vi "ISX3_Cmd_SetSetupAddFrequencyEx.vi"(1 "Use LogScale":bool, 3 "PointDelay [µs]":u32, 5 "Start Frequency [Hz]":sgl=0.01 min=0.01 max=1e+07, 7 "Stop Frequency [Hz]":sgl=0.01 min=0.01 max=1e+07, 9 "Frequency Count":sgl=1.0 min=1 max=2048 step=1, 12 "Precision":sgl min=0, 13 "Amplitude [V]":sgl=0.01 min=0.001 max=1) -> (10 "set Setup Init Cmd":u8[](array[numeric]) format="%x")   [LabVIEW 2012, in "Sciospec ISX3 Impedance Analyzer.lvlib"]
uses:
  Sciospec ISX3 Impedance Analyzer.lvlib
panel:
  in  "Use PhaseSync":bool
  # "This VI generates the command to initate a new frequency block in the system with the PhaseSync and PointDelay option"
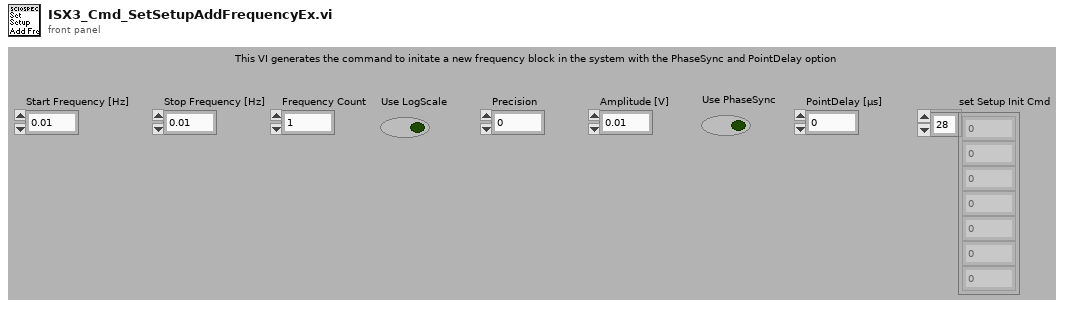
[diagram p1: front panel]
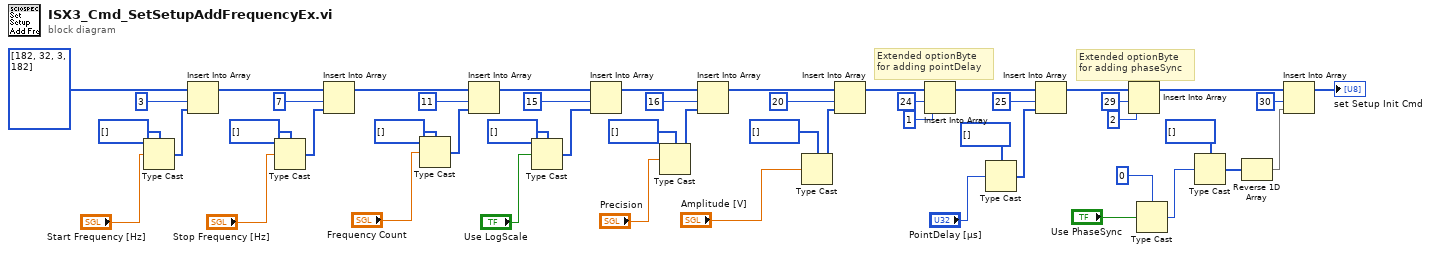
[diagram p0: block diagram]
diagram:
  # "Extended optionByte\nfor adding phaseSync"
  # "Extended optionByte\nfor adding pointDelay"
  n1 = Type Cast(type=u8[] [], x="Start Frequency [Hz]") -> (*(type *) &x=w47:u8[])
  n2 = Insert Into Array(array=u8[] [182, 32, 3, 182], index=3, new element=w47) -> (w45:u8[])
  n3 = Type Cast(type=u8[] [], x="Stop Frequency [Hz]") -> (*(type *) &x=w40:u8[])
  n4 = Insert Into Array(array=w45, index=7, new element=w40) -> (w24:u8[])
  n5 = Type Cast(type=u8[] [], x="Frequency Count") -> (*(type *) &x=w26:u8[])
  n6 = Insert Into Array(array=w24, index=11, new element=w26) -> (w23:u8[])
  n7 = Type Cast(type=u8[] [], x="Use LogScale") -> (*(type *) &x=w37:u8[])
  n8 = Insert Into Array(array=w23, index=15, new element=w37) -> (w44:u8[])
  n9 = Type Cast(type=u8[] [], x="Precision") -> (*(type *) &x=w34:u8[])
  n10 = Insert Into Array(array=w44, index=16, new element=w34) -> (w43:u8[])
  n11 = Type Cast(type=u8[] [], x="Amplitude [V]") -> (*(type *) &x=w30:u8[])
  n12 = Insert Into Array(array=w43, index=20, new element=w30) -> (w20:u8[])
  n13 = Insert Into Array(array=w20, index=24 ("Index"), new element=u8 1 ("Neues Element/Teil-Array")) -> (w10:u8[])
  n14 = Type Cast(type=u8[] [], x="PointDelay [µs]") -> (*(type *) &x=w8:u8[])
  n15 = Insert Into Array(array=w10, index=25 ("Index"), new element=w8) -> (w6:u8[])
  n16 = Insert Into Array(array=w6, index=29 ("Index"), new element=u8 2 ("Neues Element/Teil-Array")) -> (w15:u8[])
  n17 = Type Cast(type=u32 0, x="Use PhaseSync") -> (*(type *) &x=w3:u32)
  n18 = Type Cast(type=u8[] [], x=w3) -> (*(type *) &x=w2:u8[])
  n19 = Reverse 1D Array(array=w2) -> (reversed array=w1:u8[])
  n20 = Insert Into Array(array=w15, index=30 ("Index"), new element=w1) -> (→"set Setup Init Cmd":u8[])
